vi "Util Hex String to Decimal.vi"(8 "error in (no error)":errorcluster, 11 "String":string) -> (0 "error out":errorcluster, 3 "Numeric":u32)   [LabVIEW 2017, in "xHelper.lvlib"]
uses:
  xHelper.lvlib
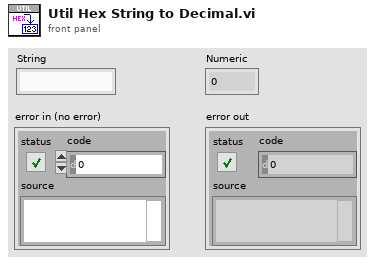
[diagram p1: front panel]
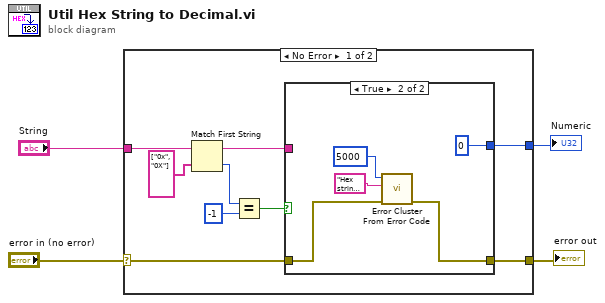
[diagram p0: block diagram]
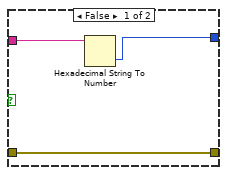
[diagram p2: hidden frame]
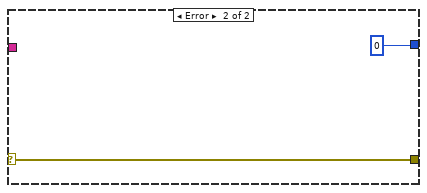
[diagram p3: hidden frame]
diagram:
  n1 = case shown="No Error" "error in (no error)" {
    selector: "error in (no error)" -> [w8 w23]
    tunnel: [w7 w23] -> w3
    tunnel: "String" -> [w13 _]
    tunnel: [w6 u32 0] -> w1
    frame No Error {
      n2 = Match First String(2:string[] ["0x", "0X"] ("string array"), 3:w13) -> (0:w11:i32, 1:w5:string)
      n3 = Equal?(x=w11, y=-1) -> (x = y?=w9:bool)
      n4 = case shown="True" w9 {
        tunnel: w8 -> [w16 w20]
        tunnel: [w16 w19] -> w7
        tunnel: [w14 u32 0] -> w6
        tunnel: w5 -> [w15 _]
        frame False {
          n5 = Hexadecimal String To Number(string=w15) -> (number=w14:u32)  [unwired: 2 in, 1 out]
        }
        frame True {
          n6 = call <vilib>:"Error Cluster From Error Code.vi"("error in (no error)"=w20, "error message (\"\")"="Hex string format is wrong!" ("error message (\"\")"), "error code (0)"=5000) -> ("error out"=w19:errorcluster)  [unwired: 6 in]
        }
      }
    }
    frame Error {
    }
  }
  "error out" <- w3
  "Numeric" <- w1
